vi "Connection.vi"(9 "?":bool, 10 "Utilisateur":string, 11 "Mot_de_passe":string) -> (3 "Boolean":bool)   [LabVIEW 2018]
uses:
  <vilib>/addons/database/Connection.llb/DB Tools Open Connec (Path).vi
  <vilib>/addons/database/Connection.llb/Conn Execute.vi
  <vilib>/addons/database/Recordset.llb/Rec Get Recordset Properties (R).vi
  <vilib>/addons/database/Recordset.llb/Rec Fetch Recordset Data (R).vi
  <vilib>/addons/database/_DB Variant To Data/Database Variant To Data.xnode
  <vilib>/addons/database/NI_Database_API.lvlib
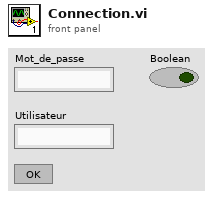
[diagram p1: front panel]
types:
  T1 = typedef "NI_Database_API.lvlib/Conn ObjectReference.ctl" = refnum<k1>
  T2 = typedef "NI_Database_API.lvlib/Rec ObjectReference.ctl" = refnum<k1>
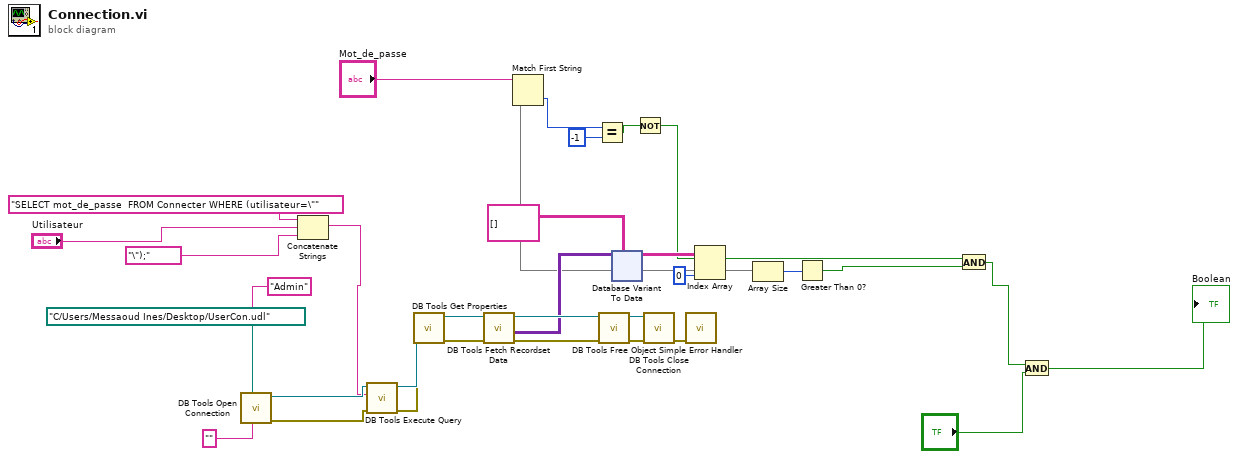
[diagram p0: block diagram]
diagram:
  n1 = call-poly <vilib>:"DB Tools Open Connection.vi"("password"="", "userID"="Admin", "connection information"=path "C:/Users/Messaoud Ines/Desktop/UserCon.udl") -> ("error out"=w24:errorcluster, "connection reference"=w9:T1)  [unwired: 5 in]
  n2 = Concatenate Strings("SELECT mot_de_passe  FROM Connecter WHERE (utilisateur=\"", "Utilisateur", "\");") -> (w8:string)
  n3 = call-poly <vilib>:"DB Tools Execute Query.vi"("error in (no error)"=w24, "SQL query"=w8, "connection reference"=w9) -> ("error out"=w23:errorcluster, "recordset reference"=w25:T2)  [unwired: 5 in]
  n4 = call-poly <vilib>:"DB Tools Get Properties.vi"("error in (no error)"=w23, "recordset reference"=w25) -> ("error out"=w30:errorcluster, "recordset reference out"=w29:T2)  [unwired: 3 in, 1 out]
  n5 = call-poly <vilib>:"DB Tools Fetch Recordset Data.vi"("error in (no error)"=w30, "recordset reference"=w29) -> ("error out"=w27:errorcluster, "recordset data"=w19:variant[][], "recordset reference out"=w28:T2)  [unwired: 3 in]
  n6 = call-poly <vilib>:"DB Tools Free Object.vi"("error in (no error)"=w27, "recordset reference"=w28) -> ("error out"=w21:errorcluster, "connection reference"=w22:T1)  [unwired: 8 in]
  n7 = xnode "Database Variant To Data"("database variant"=w19, "type"=string[][] []) -> ("data"=w17:string[][])  [unwired: 1 in, 1 out]
  n8 = call <vilib>:"DB Tools Close Connection.vi"("error in (no error)"=w21, "connection reference"=w22) -> ("error out"=w20:errorcluster)  [unwired: 5 in]
  n9 = call <vilib>:"Simple Error Handler.vi"("error in (no error)"=w20) -> ()  [unwired: 4 in, 5 out]
  n10 = Index Array(array=w17, index (col)=0 ("disabled index (col)")) -> (element=w6:string[])  [unwired: 1 in]
  n11 = Match First String(2:w6, 3:"Mot_de_passe") -> (0:w5:i32)  [unwired: 1 out]
  n12 = Equal?(x=w5, y=-1) -> (x = y?=w2:bool)
  n13 = Not(x=w2) -> (.not. x?=w3:bool)
  n14 = Array Size(array=w6) -> (size(s)=w15:i32)
  n15 = Greater Than 0?(x=w15) -> (x > 0?=w1:bool)
  n16 = And(x=w3, y=w1) -> (x .and. y?=w31:bool)
  n17 = And(x=w31, y="?") -> (x .and. y?=→"Boolean":bool)
